vi "Open.vi"(4 "Permissions":T2={"Owner"={"Read"=TRUE, "Write"=TRUE, "Execute"=FALSE}, "Group"={"Read"=TRUE, "Write"=FALSE, "Execute"=FALSE}, "Others"={"Read"=TRUE, "Write"=FALSE, "Execute"=FALSE}}, 6 "Flags":T1={"Read"=TRUE, "Write"=TRUE, "Append"=FALSE, "Create"=FALSE, "Truncate"=FALSE, "Exclude"=FALSE}, 8 "Error In":errorcluster, 10 "Remote Path":string, 11 "SFTP":refnum<class "SFTP.lvclass">) -> (0 "Error Out":errorcluster, 3 "SFTP File":refnum<class "SFTP File.lvclass">)   [LabVIEW 2018, in "Toolkit.lvlib" / "SFTP File.lvclass"]
uses:
  SFTP File.lvclass
  SFTP/SFTP.lvclass
  Type Definitions/Permissions.ctl
  Type Definitions/Modes.ctl
  Type Definitions/Flags.ctl
  SFTP/SFTP.lvclass/SFTP.ctl
  Session/Session.lvclass/Session.ctl
  SSH/SSH.lvclass/SSH.ctl
  SFTP File.lvclass/SFTP File.ctl
  Toolkit.lvlib
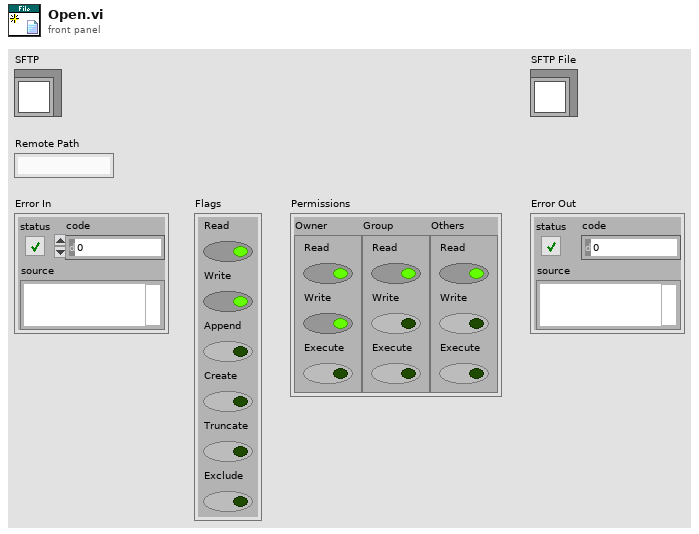
[diagram p1: front panel]
types:
  T1 = typedef "Toolkit.lvlib/SFTP File.lvclass/Flags.ctl" = cluster{"Read":bool, "Write":bool, "Append":bool, "Create":bool, "Truncate":bool, "Exclude":bool}
  T2 = typedef "Toolkit.lvlib/Permissions.ctl" = cluster{"Owner":T3, "Group":T3, "Others":T3}
  T3 = typedef "Toolkit.lvlib/Modes.ctl" = cluster{"Read":bool, "Write":bool, "Execute":bool}
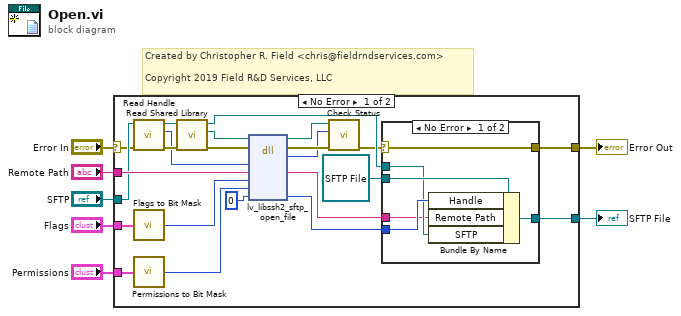
[diagram p0: block diagram]
diagram:
  # "Created by Christopher R. Field <chris@fieldrndservices.com>\n\nCopyright 2019 Field R&D Services, LLC"
  n1 = case shown="No Error" "Error In" {
    selector: "Error In" -> [w24 w39]
    tunnel: [w9 w39] -> w6
    tunnel: "SFTP" -> [w25 _]
    tunnel: "Remote Path" -> [w30 _]
    tunnel: [w17 _] -> w3
    tunnel: "Permissions" -> [w16 _]
    tunnel: "Flags" -> [w14 _]
    frame No Error {
      n2 = call "Read Handle.vi"("Error In"=w24, "SFTP In"=w25) -> ("Erorr Out"=w22:errorcluster, "Handle"=w21:u64, "SFTP Out"=w23:refnum<class "SFTP.lvclass">)  [unwired: 7 in]
      n3 = call "Flags to Bit Mask.vi"("Flags"=w14) -> ("Bit Mask"=w13:u32)
      n4 = call "Permissions to Bit Mask.vi"("Permissions"=w16) -> ("Bit Mask"=w15:u32)
      n5 = call "Read Shared Library.vi"("Error In"=w22, "SFTP In"=w23) -> ("Erorr Out"=w20:errorcluster, "libssh2lv Shared Library"=w11:path, "SFTP Out"=w12:refnum<class "SFTP.lvclass">)  [unwired: 7 in]
      n6 = dll-call lib="D:/Users/cfield/Code/Field R&D Services/SSH/LV-LIBSSH2/LabVIEW/trunk/src/Toolkit/Support/lv-libssh2.*" fn="lv_libssh2_sftp_open_file"(path in=w11, error in=w20, "sftp"=w21, "path"=w30, "flags"=w13, "permissions"=w15, "handle"=u64 0) -> (path out=w29:path, error out=w28:errorcluster, "status"=w27:i32, "path"=w8:string, "handle"=w18:u64)  [unwired: 4 in]
      n7 = call "Check Status.vi"("Error In"=w28, "Status"=w27, "lv-libssh2 Shared Library In"=w29) -> ("Error Out"=w10:errorcluster)  [unwired: 7 in, 1 out]
      n8 = case shown="No Error" w10 {
        selector: w10 -> [w32 w37]
        tunnel: refnum<class "SFTP File.lvclass"> refnum ("Toolkit.lvlib:SFTP File.lvclass") -> [w36 w38]
        tunnel: w18 -> [w35 _]
        tunnel: [w34 w38] -> w17
        tunnel: w12 -> [w33 _]
        tunnel: [w32 w37] -> w9
        tunnel: w8 -> [w31 _]
        frame No Error {
          n9 = Bundle By Name(cluster=w36, "Handle"=w35, "Remote Path"=w31, "SFTP"=w33) -> (w34:refnum<class "SFTP File.lvclass">)
        }
        frame Error {
        }
      }
    }
    frame Error {
    }
  }
  "Error Out" <- w6
  "SFTP File" <- w3
